vi "(SubVI)Launcher_Error Log.vi"(8 "error in (no error)":errorcluster caption="에러 입력(에러 없음)", 10 "Previous State":T1, 11 "Error State":T1) -> (0 "error out":errorcluster caption="에러 출력")   [LabVIEW 2020]
uses:
  Controls/(Ctrl)Launcher_State Machine.ctl
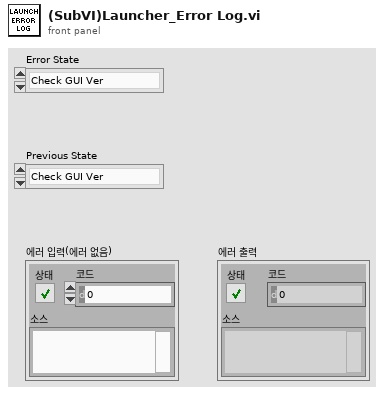
[diagram p1: front panel]
types:
  T1 = typedef "(Ctrl)Launcher_State Machine.ctl" = enum16{"Check GUI Ver", "Update GUI", "Connect to BD", "Check FW Ver", "Update FW", "Check Edition", "Launch", "Server Connection Error", "BD Connection Error", "FW Update Error"}
  T2 = enum16{"open", "replace", "create", "open or create", "replace or create", "replace or create with confirmation"}
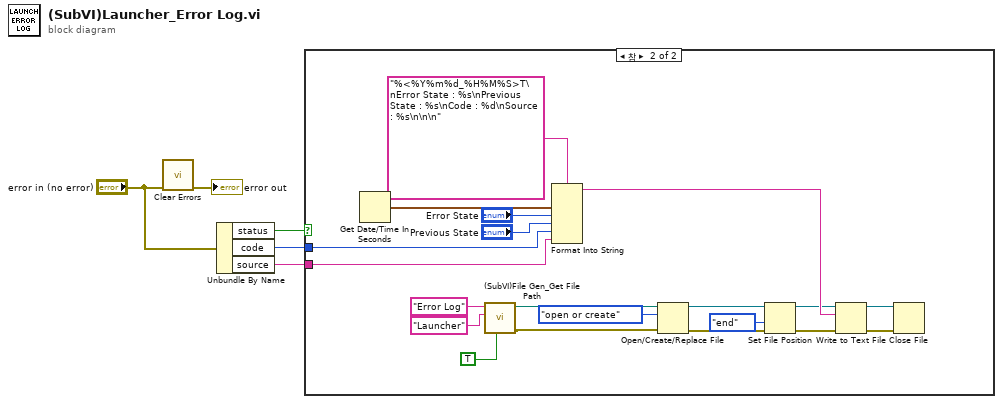
[diagram p0: block diagram]
diagram:
  n1 = call <vilib>:"Clear Errors.vi"("error in (no error)"="error in (no error)") -> ("error out"=→"error out":errorcluster)  [unwired: 5 in, 1 out]
  n2 = Unbundle By Name("error in (no error)") -> ("status"=w3:bool, "code"=w2:i32, "source"=w1:string)
  n3 = case shown="참" w3 {
    tunnel: w2 -> [_ w22]
    tunnel: w1 -> [_ w23]
    frame False {
    }
    frame True {
      n4 = Get Date/Time In Seconds() -> (seconds since 1Jan1904=w25:timestamp)
      n5 = call "(SubVI)File Gen_Get File Path.vi"("Common?"=TRUE, "File Name"="Launcher", "Folder Name"="Error Log") -> ("error out"=w15:errorcluster, "Path"=w17:path)  [unwired: 6 in, 1 out]
      n6 = Format Into String(format string="%<%Y%m%d_%H%M%S>T\nError State : %s\nPrevious State : %s\nCode : %d\nSource : %s\n\n\n" ("포맷 문자열"), w25, "Error State", "Previous State", w22, w23) -> (resulting string=w13:string)  [unwired: 2 in, 1 out]
      n7 = Open/Create/Replace File(file path (use dialog)=w17, error in=w15, operation (0:open)=T2."open or create" ("동작(0:open)")) -> (refnum out=w9:refnum<file>, error out=w14:errorcluster)  [unwired: 3 in, 1 out]
      n8 = Set File Position(refnum=w9, from (0:start)=enum16{"start", "end", "current"}."end" ("위치(0:start)"), error in=w14) -> (refnum out=w8:refnum<file>, error out=w10:errorcluster)  [unwired: 1 in]
      n9 = Write to Text File(file (use dialog)=w8, text=w13, error in=w10) -> (refnum out=w12:refnum<file>, error out=w11:errorcluster)  [unwired: 1 in, 1 out]
      n10 = Close File(refnum=w12, error in=w11) -> ()  [unwired: 2 out]
    }
  }
